vi "ASCII Intermittent Instrument.vi"() -> ()   [LabVIEW 2019]
uses:
  <vilib>/numeric/Random Number (Range) DBL.vi
  <vilib>/Instr/_visa.llb/VISA Configure Serial Port (Instr).vi
panel:
  in  "Send":bool
  out "read buffer":string
  out "error out":errorcluster
  in  "stop":bool
  in  "VISA resource name":refnum<visa-resource-name>
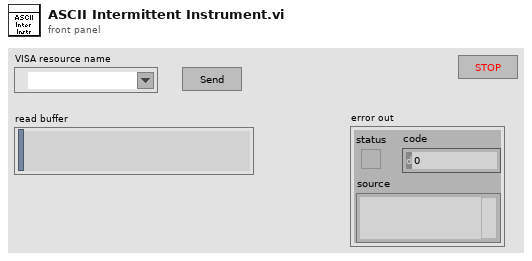
[diagram p1: front panel]
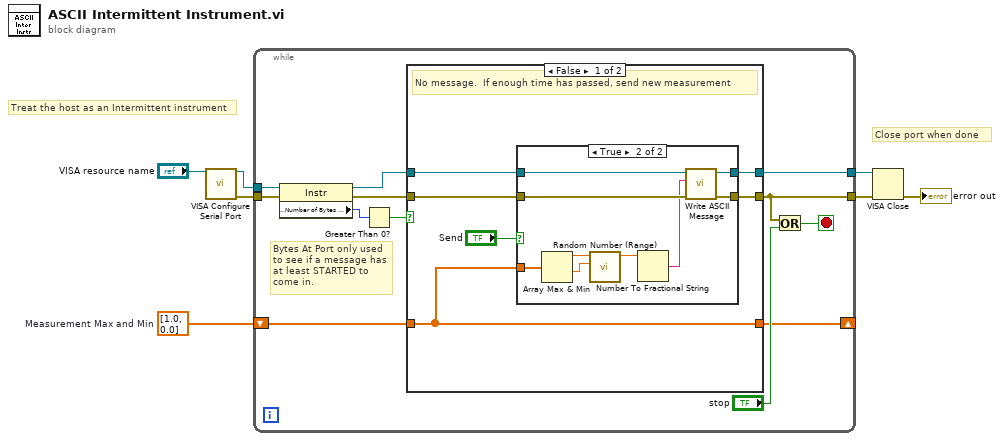
[diagram p0: block diagram]
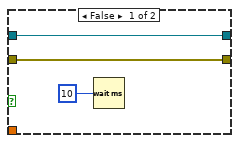
[diagram p2: hidden frame]
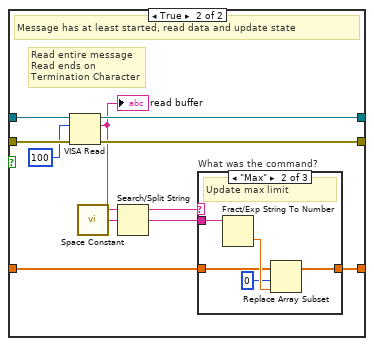
[diagram p3: hidden frame]
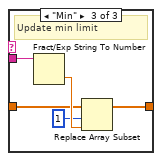
[diagram p5: hidden frame]
diagram:
  w2 = dbl[] [1.0, 0.0]  # Measurement Max and Min
  # "Treat the host as an Intermittent instrument"
  # "Close port when done"
  n1 = call-poly "VISA Configure Serial Port"("VISA resource name"="VISA resource name") -> ("VISA resource name out"=w1:refnum<visa-resource-name>, "error out"=w5:errorcluster)  [unwired: 13 in]
  n2 = while {
    tunnel: w5 -> [w19]
    tunnel: w1 -> [w16]
    tunnel: [w12] -> w3
    tunnel: [w17] -> w7
    shift-right: [w8] -> _
    shift-left: w2 -> [w9]
    stop <- w11 stop-if-true
    # "Bytes At Port only used\nto see if a message has\nat least STARTED to\ncome in."
    n3 = property class="Instr"(reference=w16, error in=w19) -> (reference out=w13:refnum<visa-resource-name>, error out=w18:errorcluster, "Serial Settings:Number of Bytes at Serial Port"=w15:u32)
    n4 = Greater Than 0?(x=w15) -> (x > 0?=w14:bool)
    n5 = case shown="False" w14 {
      tunnel: w18 -> [w25 w48]
      tunnel: w13 -> [w23 w46]
      tunnel: [w21 w44] -> w12
      tunnel: [w24 w47] -> w17
      tunnel: w9 -> [w22 w39]
      tunnel: [w22 w38] -> w8
      frame False {
        # "No message.  If enough time has passed, send new measurement"
        n6 = case shown="True" "Send" {
          tunnel: w23 -> [w27 w31]
          tunnel: w25 -> [w28 w37]
          tunnel: w22 -> [_ w35]
          tunnel: [w27 w30] -> w21
          tunnel: [w28 w36] -> w24
          frame False {
            n7 = Wait (ms)(milliseconds to wait=u32 10) -> ()  [unwired: 1 out]
          }
          frame True {
            n8 = Array Max & Min(array=w35) -> (max value=w34:dbl, min value=w33:dbl)  [unwired: 2 out]
            n9 = call-poly <vilib>:"Random Number (Range).vi"("lower bound (0)"=w33, "upper bound (100)"=w34) -> ("number"=w32:dbl)  [unwired: 9 in]
            n10 = Number To Fractional String(number=w32) -> (F-format string=w29:string)  [unwired: 3 in]
            n11 = call "Write ASCII Message.vi"("error in"=w37, "Message"=w29, "VISA resource in"=w31) -> ("error out"=w36:errorcluster, "VISA resource out"=w30:refnum<visa-resource-name>)  [unwired: 7 in]
          }
        }
      }
      frame True {
        # "Read entire message\nRead ends on\nTermination Character"
        # "Message has at least started, read data and update state"
        n12 = VISA Read(VISA resource name=w46, byte count=u32 100, error in (no error)=w48) -> (VISA resource name out=w44:refnum<visa-resource-name>, read buffer=w43:string, error out=w47:errorcluster)  [unwired: 1 out]
        "read buffer" <- w43
        n13 = call <vilib>:"Space Constant.vi"() -> ("String"=w42:string)
        n14 = Search/Split String(string=w43, search string/char (-)=w42) -> (substring before match=w41:string, match + rest of string=w40:string)  [unwired: 1 in, 1 out]
        n15 = case "What was the command?" shown="\"Max\"" w41 {
          tunnel: w40 -> [_ w53 w58]
          tunnel: w39 -> [w49 w52 w57]
          tunnel: [w49 w50 w55] -> w38
          frame Default {
            # "Unknown command"
          }
          frame "Max" {
            # "Update max limit"
            n16 = Fract/Exp String To Number(string=w53) -> (number=w54:dbl)  [unwired: 3 in, 1 out]
            n17 = Replace Array Subset(array=w52, new element=w54, index=0) -> (w50:dbl[])
          }
          frame "Min" {
            # "Update min limit"
            n18 = Fract/Exp String To Number(string=w58) -> (number=w59:dbl)  [unwired: 3 in, 1 out]
            n19 = Replace Array Subset(array=w57, new element=w59, index=1) -> (w55:dbl[])
          }
        }
      }
    }
    n20 = Or(x=w17, y="stop") -> (x .or. y?=w11:bool)
  }
  n21 = VISA Close(VISA resource name=w3, error in (no error)=w7) -> (error out=→"error out":errorcluster)
